vi "local-var-example.vi"() -> ()   [LabVIEW 2012]
panel:
  out "Chart-1":dbl(graph)
  in  "ONOFF SWITCH":bool=TRUE
  out "Chart-2":dbl(graph)
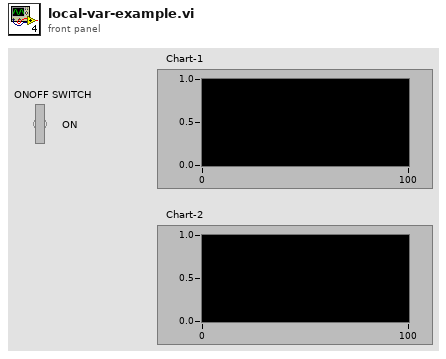
[diagram p1: front panel]
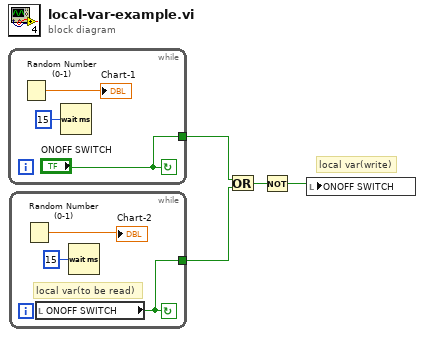
[diagram p0: block diagram]
diagram:
  # "local var(write)"
  n1 = while {
    tunnel: ["ONOFF SWITCH"] -> w3
    stop <- "ONOFF SWITCH" continue-if-true
    n2 = Random Number (0-1)() -> (number: 0 to 1=→"Chart-1":dbl)
    n3 = Wait (ms)(milliseconds to wait=u32 15) -> ()  [unwired: 1 out]
  }
  n4 = while {
    tunnel: [w9] -> w2
    stop <- w9 continue-if-true
    # "local var(to be read)"
    n5 = Random Number (0-1)() -> (number: 0 to 1=→"Chart-2":dbl)
    n6 = local read "ONOFF SWITCH"() -> (w9:bool)
    n7 = Wait (ms)(milliseconds to wait=u32 15) -> ()  [unwired: 1 out]
  }
  n8 = Or(x=w3, y=w2) -> (x .or. y?=w4:bool)
  n9 = Not(x=w4) -> (.not. x?=w1:bool)
  n10 = local write "ONOFF SWITCH"(w1) -> ()
